vi "GLLL_Test1.vi"() -> ()   [LabVIEW 2014]
uses:
  ListHead.lvclass
panel:
  out "ResIndex":i32
  out "PopedContent2":u32
  out "IncArray":i32[](array[numeric])
  out "PopedContent":u32
  out "DecArray":i32[](array[numeric])
  out "OutputArray":i32[](array[numeric])
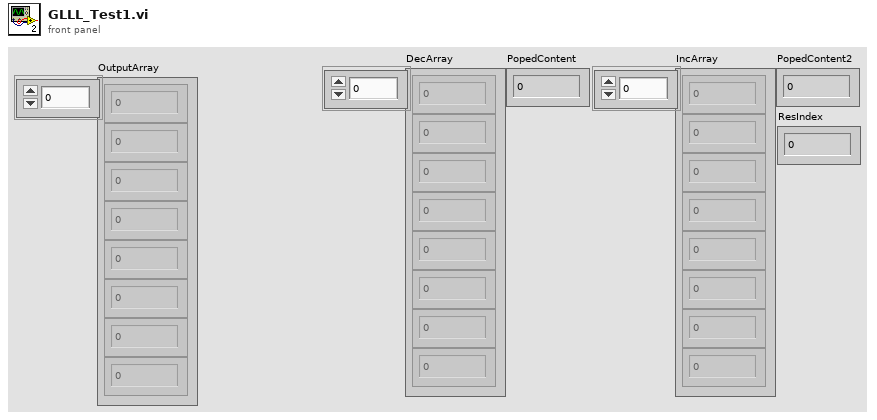
[diagram p1: front panel]
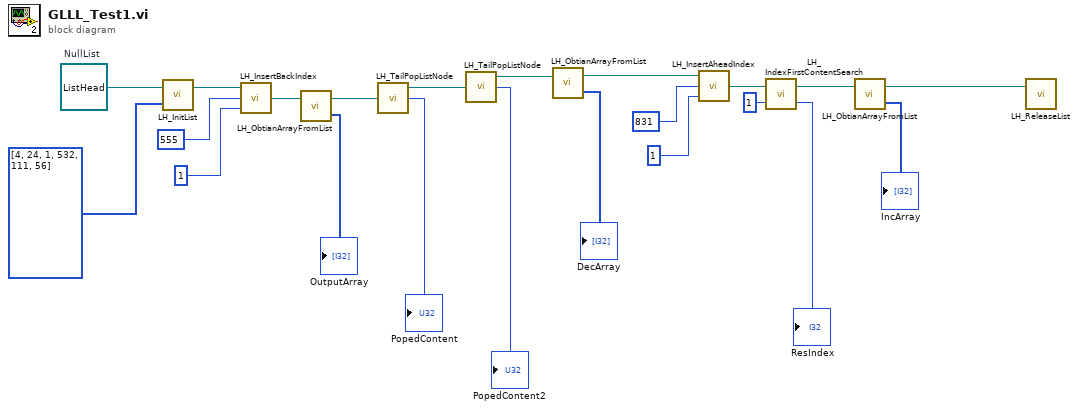
[diagram p0: block diagram]
diagram:
  w22 = refnum<class "ListHead.lvclass"> refnum  # NullList
  n1 = call "LH_InitList.vi"("InputContents"=i32[] [4, 24, 1, 532, 111, 56], "InputList"=w22) -> ("OutputList"=w19:refnum<class "ListHead.lvclass">)  [unwired: 1 in]
  n2 = call "LH_InsertBackIndex.vi"("Index"=1, "InsertContent"=555, "InputList"=w19) -> ("OutputList"=w18:refnum<class "ListHead.lvclass">)
  n3 = call "LH_ObtianArrayFromList.vi"("InputList"=w18) -> ("OutputArray"=→"OutputArray":i32[], "OutputList"=w15:refnum<class "ListHead.lvclass">)  [unwired: 1 in]
  n4 = call "LH_TailPopListNode.vi"("InputList"=w15) -> ("OutputList"=w7:refnum<class "ListHead.lvclass">, "Content"=→"PopedContent":u32)  [unwired: 1 out]
  n5 = call "LH_TailPopListNode.vi"("InputList"=w7) -> ("OutputList"=w8:refnum<class "ListHead.lvclass">, "Content"=→"PopedContent2":u32)  [unwired: 1 out]
  n6 = call "LH_ObtianArrayFromList.vi"("InputList"=w8) -> ("OutputArray"=→"DecArray":i32[], "OutputList"=w12:refnum<class "ListHead.lvclass">)  [unwired: 1 in]
  n7 = call "LH_InsertAheadIndex.vi"("Index"=1, "InsertContent"=831, "InputList"=w12) -> ("OutputList"=w5:refnum<class "ListHead.lvclass">)
  n8 = call "LH_IndexFirstContentSearch.vi"("TargetContent"=1, "InputList"=w5) -> ("ResIndex"=→"ResIndex":i32, "Output"=w2:refnum<class "ListHead.lvclass">)
  n9 = call "LH_ObtianArrayFromList.vi"("InputList"=w2) -> ("OutputArray"=→"IncArray":i32[], "OutputList"=w1:refnum<class "ListHead.lvclass">)  [unwired: 1 in]
  n10 = call "LH_ReleaseList.vi"("InputList"=w1) -> ()  [unwired: 3 in]
